vi "eat.vi"(0 "reference in":refnum<class "Parent.lvclass">, 5 "error in (no error)":errorcluster) -> (14 "reference out":refnum<class "Parent.lvclass">, 19 "error out":errorcluster)   [LabVIEW 2019, in "Parent.lvclass"]
uses:
  Parent.lvclass
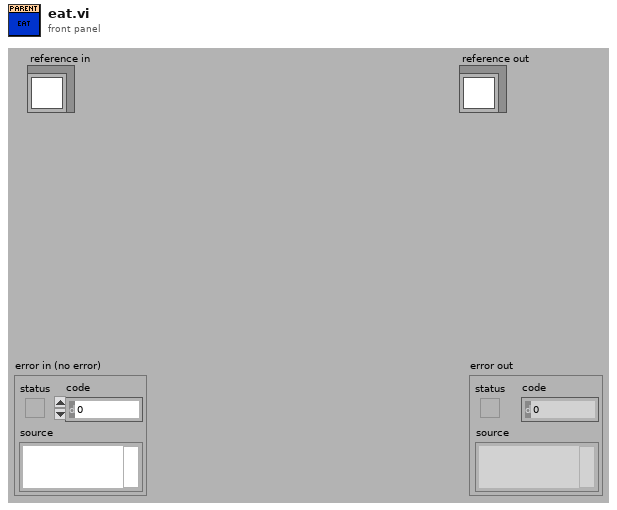
[diagram p1: front panel]
types:
  T1 = typedef "Parent.lvclass/ObjectAttributes.ctl" = cluster{"ParentAttribute":dbl}
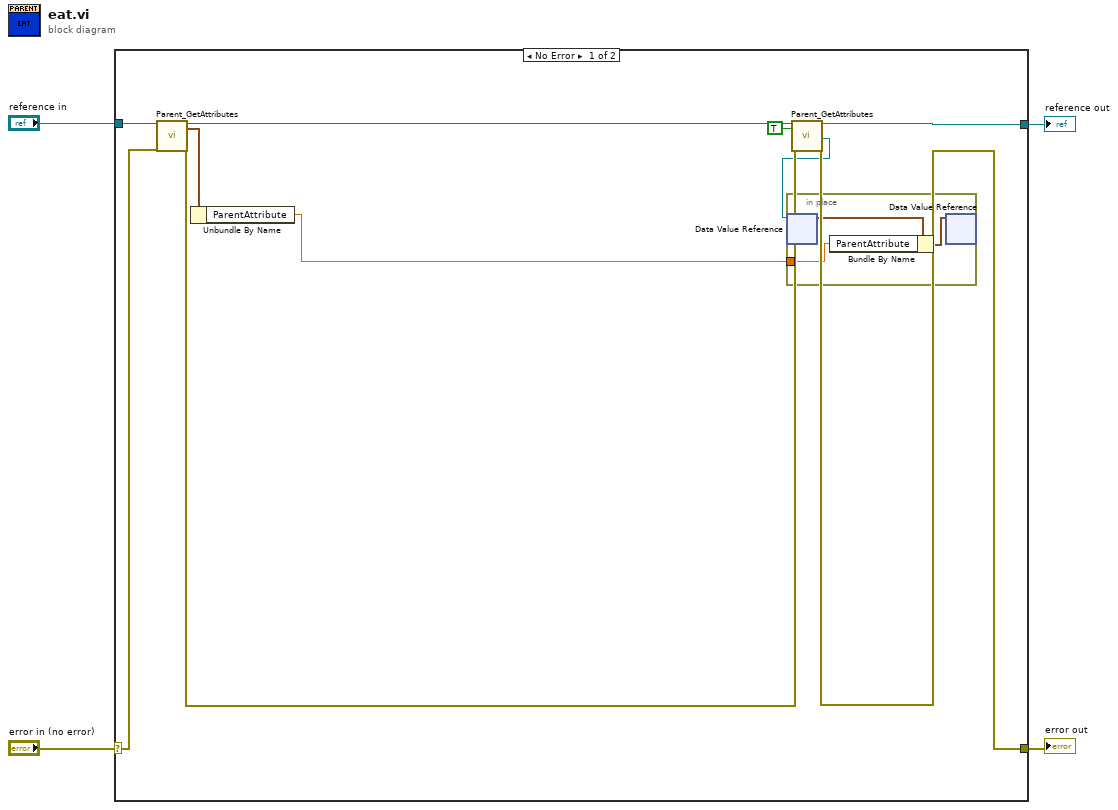
[diagram p0: block diagram]
diagram:
  n1 = case shown="No Error" "error in (no error)" {
    selector: "error in (no error)" -> [w11 w19]
    tunnel: [w14 w19] -> w3
    tunnel: [w13 w18] -> w1
    tunnel: "reference in" -> [w12 w18]
    frame No Error {
      n2 = call "Parent_GetAttributes.vi"("reference in"=w12, "error in (no error)"=w11) -> ("reference out"=w9:refnum<class "Parent.lvclass">, "Data"=w7:T1, "error out"=w10:errorcluster)  [unwired: 14 in, 1 out]
      n3 = Unbundle By Name(w7) -> ("ParentAttribute"=w5:dbl)
      n4 = call "Parent_GetAttributes.vi"("reference in"=w9, "OnlyGetDvrReference(False)"=TRUE, "error in (no error)"=w10) -> ("reference out"=w13:refnum<class "Parent.lvclass">, "DataRef"=w6:refnum<data-value>, "error out"=w14:errorcluster)  [unwired: 13 in, 1 out]
      n5 = in-place {
        in-place-border: w5 -> [w16]
        n6 = in-place-dvr #1(w6) -> (w17:T1)  [unwired: 1 out]
        n7 = Bundle By Name(cluster=w17, "ParentAttribute"=w16) -> (w15:T1)
        n8 = in-place-dvr #1(w15) -> ()  [unwired: 2 out]
      }
    }
    frame Error {
    }
  }
  "error out" <- w3
  "reference out" <- w1
